vi "LED ON_OFF.vi"() -> ()   [LabVIEW 2014]
panel:
  in  "stop":bool
  in  "Boolean 2":bool
  out "Boolean":bool
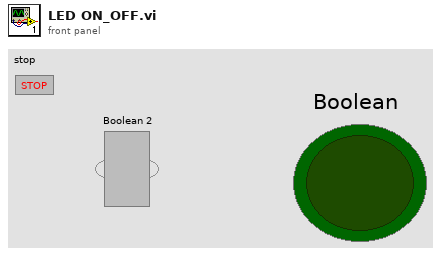
[diagram p1: front panel]
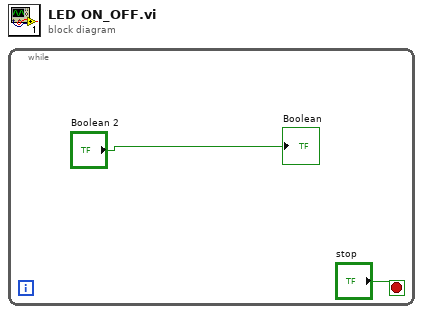
[diagram p0: block diagram]
diagram:
  n1 = while {
    stop <- "stop" stop-if-true
    "Boolean" <- "Boolean 2"
  }
